vi "DSA Stop AI and AO.vi"(0 "Task ID Cluster":T1, 5 "error in":errorcluster, 10 "Buffer Complete":bool, 12 "WT Errors In":errorcluster) -> (14 "AI Task ID Out":refnum<k21>, 15 "AO Task ID Out":refnum<k21>[](array[refnum]), 19 "errors out":errorcluster)   [LabVIEW 2021]
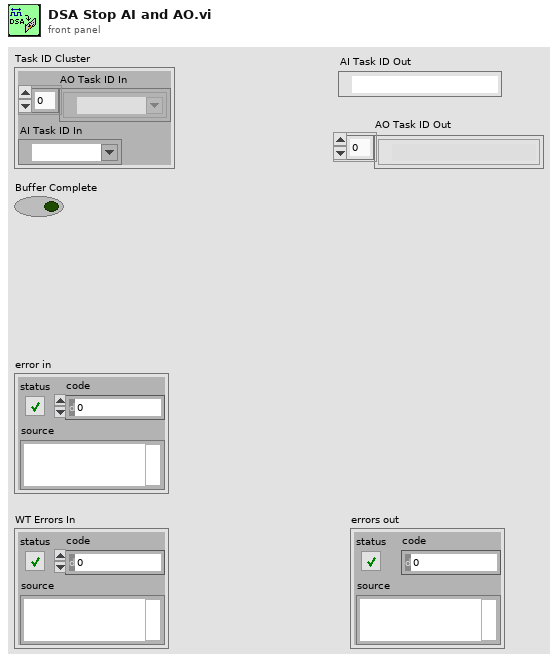
[diagram p1: front panel]
types:
  T1 = cluster{"AO Task ID In":refnum<k21>[], "AI Task ID In":refnum<k21>}
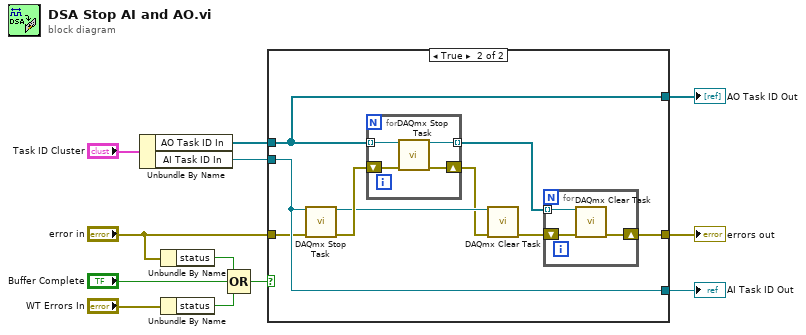
[diagram p0: block diagram]
diagram:
  n1 = Unbundle By Name("Task ID Cluster") -> ("AO Task ID In"=w9:refnum<k21>[], "AI Task ID In"=w8:refnum<k21>)
  n2 = Unbundle By Name("error in") -> ("status"=w6:bool)
  n3 = Unbundle By Name("WT Errors In") -> ("status"=w5:bool)
  n4 = Compound Arithmetic op=OR(w6, "Buffer Complete", w5) -> (w7:bool)
  n5 = case shown="True" w7 {
    tunnel: w9 -> [w15 w24]
    tunnel: w8 -> [w14 w23]
    tunnel: "error in" -> [w13 w22]
    tunnel: [w13 w16] -> w1
    tunnel: [w15 w24] -> w11
    tunnel: [w14 w23] -> w2
    frame False {
    }
    frame True {
      n6 = call <vilib>:"DAQmx Stop Task.vi"("task/channels in"=w23, "error in"=w22) -> ("task out"=w20:refnum<k21>, "error out"=w21:errorcluster)  [unwired: 12 in]
      n7 = for {
        tunnel: w24 -> [w31] mode=indexing
        shift-right: [w29] -> w19
        shift-left: w21 -> [w30]
        tunnel: [w28] -> w17 mode=indexing
        n8 = call <vilib>:"DAQmx Stop Task.vi"("task/channels in"=w31, "error in"=w30) -> ("task out"=w28:refnum<k21>, "error out"=w29:errorcluster)  [unwired: 12 in]
      }
      n9 = call <vilib>:"DAQmx Clear Task.vi"("task in"=w20, "error in"=w19) -> ("error out"=w18:errorcluster)  [unwired: 13 in]
      n10 = for {
        shift-right: [w27] -> w16
        shift-left: w18 -> [w26]
        tunnel: w17 -> [w25] mode=indexing
        n11 = call <vilib>:"DAQmx Clear Task.vi"("task in"=w25, "error in"=w26) -> ("error out"=w27:errorcluster)  [unwired: 13 in]
      }
    }
  }
  "AO Task ID Out" <- w11
  "AI Task ID Out" <- w2
  "errors out" <- w1
